vi "State to Context.vi"(7 "Context in (for Preserve Run-Time Class)":refnum<class "State Pattern.lvclass">, 8 "error in":errorcluster, 11 "State in":refnum<class "State Pattern.lvclass">) -> (0 "error out":errorcluster, 2 "Context out":refnum<class "State Pattern.lvclass">)   [LabVIEW 2021, in "State Pattern.lvclass"]
uses:
  State Pattern.lvclass
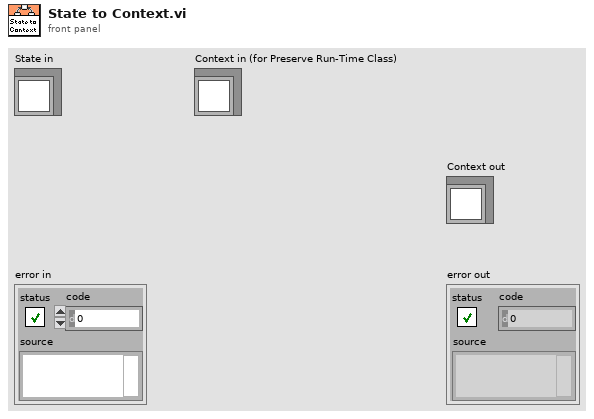
[diagram p1: front panel]
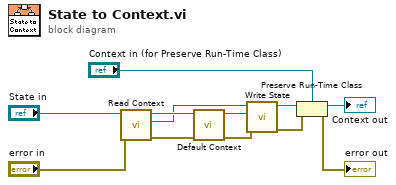
[diagram p0: block diagram]
diagram:
  n1 = call-dynamic "Read Context.vi"("error in"="error in", "State in"="State in") -> ("error out"=w1:errorcluster, "Context"=w2:refnum<class "State Pattern.lvclass">, "State out"=w3:refnum<class "State Pattern.lvclass">)  [unwired: 7 in]
  n2 = call "Default Context.vi"("error in"=w1, "State in"=w3) -> ("error out"=w6:errorcluster, "State out"=w10:refnum<class "State Pattern.lvclass">)  [unwired: 8 in]
  n3 = call-dynamic "Write State.vi"("error in"=w6, "State"=w10, "Context in"=w2) -> ("error out"=w12:errorcluster, "Context out"=w11:refnum<class "State Pattern.lvclass">)  [unwired: 7 in]
  n4 = Preserve Run-Time Class(object in=w11, error in=w12, 2:"Context in (for Preserve Run-Time Class)") -> (object out=→"Context out":refnum<class "State Pattern.lvclass">, error out=→"error out":errorcluster)
